vi "Dashboard Main_1366_768.vi"() -> ()   [LabVIEW 2020]
uses:
  ArmGamePiecePreset.ctl
  ArmPositionPreset.ctl
  <vilib>/Rock Robotics/WPI/ThirdParty/JAS_Junk/TrajLib/TypeDef/FieldDisp_ElementPicture.ctl
  <vilib>/Rock Robotics/WPI/Solenoid/WPI_SolenoidValue.ctl
  <vilib>/event_ctls.llb/eventvkey.ctl
  <vilib>/Rock Robotics/WPI/ThirdParty/JAS_Junk/TrajLib/Rotation2d_CreateAngle.vi
  <vilib>/Rock Robotics/WPI/ThirdParty/JAS_Junk/TrajLib/Translation2d_Create.vi
  <vilib>/Rock Robotics/WPI/ThirdParty/JAS_Junk/TrajLib/VI/FieldDisp_Element_Rotate.vi
  <vilib>/Rock Robotics/WPI/ThirdParty/JAS_Junk/TrajLib/Conv_Meters_Inches.vi
  <vilib>/Rock Robotics/WPI/ThirdParty/JAS_Junk/TrajLib/Conv_Radians_Deg.vi
  <vilib>/Rock Robotics/WPI/Dashboard/WPI_DashboardLogging Global.vi
  <vilib>/Rock Robotics/Network Tables/NT Read Boolean.vi
  <vilib>/Rock Robotics/Network Tables/NT Read Integer.vi
  <vilib>/picture/pixmap.llb/Flatten Pixmap.vi
  <vilib>/picture/pictutil.llb/Create Mask.vi
  <vilib>/picture/picture.llb/Draw Flattened Pixmap.vi
  <vilib>/Rock Robotics/WPI/ThirdParty/JAS_Junk/TrajLib/Trajectory_Library.lvlib
panel:
  out "ROBOT":T1
  out "Camera Perf":string
  in  "Camera Settings":T2={"Frame Rate"=30, "Compression"=30, "Size"=1, "DB Camera Config"=FALSE} {"Frame Rate" scale=1.0..30.0; "Compression" scale=100.0..-1.0; "Size" items=["640x480", "320x240", "160x120"]}
  in  "TCP":refnum<k5>
  in  "Rec Mode":enum32{"Stop", "Record", "Playback"}(radio)
  out "Robot IP":string
  out "Image Message":string="Timeout in Camera Communications"
  in  "Dashboard Tab":T3(tab)
  out "Double Cmd1":T4
  out "Double Cmd2":T4
  out "Single Cmd1":T4
  out "Single Cmd2":T4
  out "Request":bool
  out "On Command":bool
  out "On Command":bool
  out "Request":bool
  out "Current":dbl format="%12.2f"
  out "Running":bool
  out "Enabled":bool
  out "NT Connection":bool
  out "Mode":T5(ring)=enum."Auto Disabled"
  out "Right Camera Perf":cluster{"Bandwidth (Mbps)":dbl, "FPS":dbl}
  out "Shelf":bool
  out "Floor":bool
  out "Right April Tag Updated":bool
  out "Left April Tag Updated":bool
  out "Right Cam Connected":bool
  out "Left Cam Connected":bool
  out "Field Picture":picture
  out "Odom X Pos Ft":dbl format="%14.2f"
  out "Odom Y Pos Ft":dbl format="%14.2f"
  out "Odom Heading Deg":dbl format="%14.2f"
  in  "Distance":dbl
  in  "Position":T6=enum."Middle"
  in  "Game Piece":T7
  in  "Update":bool
  in  "Starting Heading Deg":dbl
  in  "Starting Y Ft":dbl
  in  "Starting X Ft":dbl
  in  "DB/String 9":string
  in  "DB/String 8":string
  in  "DB/String 7":string
  in  "DB/String 6":string
  in  "DB/String 5":string
  in  "DB/String 4":string
  in  "DB/String 3":string
  in  "DB/String 2":string
  in  "DB/String 1":string
  in  "DB/String 0":string
  in  "DB/Slider 0":dbl(slide) scale=0.0..5.0
  in  "DB/Slider 1":dbl(slide) scale=0.0..5.0
  in  "DB/Slider 2":dbl(slide) scale=0.0..5.0
  in  "DB/Slider 3":dbl(slide) scale=0.0..5.0
  out "DB/LED 3":bool
  out "DB/LED 2":bool
  out "DB/LED 1":bool
  out "DB/LED 0":bool
  in  "DB/Button 3":bool
  in  "DB/Button 2":bool
  in  "DB/Button 1":bool
  in  "DB/Button 0":bool caption="New Name"
  out "Compressor Chart":cluster{"value":dbl, "value":dbl, "value":dbl}(graph)
  out "Single Solenoid Chart":cluster{"value":dbl, "value":dbl, "value":dbl}(graph)
  out "Double Solenoid Chart":cluster{"value":dbl, "value":dbl, "value":dbl}(graph)
  in  "Test Slider":dbl(slide) scale=0.0..100.0 scale format="%#_3g"
  in  "On/Off":bool caption="Solenoid"
  in  "Test Name":u16(ring) items=["Select the test to run..."]
  in  "Test Tree":string(tree)
  in  "Motor":cluster{"Value":dbl, "Enable":bool} {"Value" scale=-1.0..1.0 scale format="%#_3g"}
  out "Progress":T8 {"Test Progress" scale=0.0..100.0}
  in  "Rev/Fwd":cluster{"Forward":bool, "Reverse":bool}
  in  "Test Ring":u16(ring) items=["Monochrome", "Color"]
  in  "CheckList":i32(listbox)
  out "Tree":string(tree)
  out "Camera Image":T9(plugin-control)
  out "Background":bool
  in  "Camera Name":string(combo)="No Camera Selection"
  # "HW"
  # "Double Solenoid"
  # "Single Solenoid"
  # "Compressor"
  # "Quick Auto Settings"
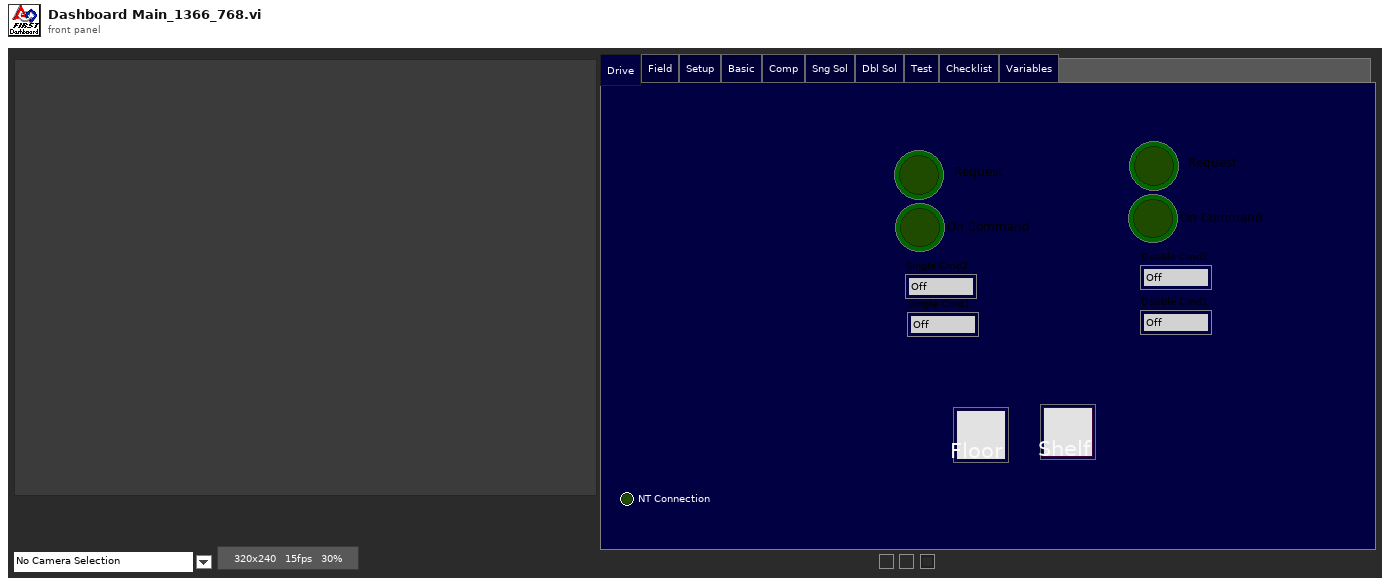
[diagram p1: front panel]
types:
  T1 = typedef "Trajectory_Library.lvlib/FieldDisp_ElementPicture.ctl" = picture
  T2 = cluster{"Frame Rate":i32, "Compression":i32, "Size":u16, "DB Camera Config":bool}
  T3 = enum32{"Drive", "Field", "Setup", "Basic", "Comp", "Sng Sol", "Dbl Sol", "Test", "Checklist", "Variables"}
  T4 = typedef "WPI_SolenoidValue.ctl" = enum16{"Off", "On", "Forward", "Reverse"}
  T5 = enum8{"Tele-Op Disabled", "Tele-Op Enabled", "Auto Disabled", "Auto Enabled", "Test Disabled", "Test Enabled", "Disconnected", "No Code", "E-Stop"}
  T6 = typedef "ArmPositionPreset.ctl" = enum16{"Upper", "Lower", "Middle", "Home", "Shelf", "Floor"}
  T7 = typedef "ArmGamePiecePreset.ctl" = enum16{"Cube", "Cone"}
  T8 = cluster{"Test Progress":u8, "Test Progress Text":string}
  T9 = typedef "IMAQ Image.ctl" = refnum<image>
  T10 = enum32{"Drive", "Field", "Setup", "Basic", "DrvLeft", "DrvRight", "ArmExtend", "ArmLift", "Bal", "Test", "Checklist", "Variables"}
  T11 = cluster{"Save Path":path, "Interval (s)":dbl, "Keep":i32}
  T12 = typedef "Image Type" = u32
  T13 = cluster{"Camera Image":refnum<vi>, "Dashboard Tab":refnum<vi>, "Background":refnum<vi>, "Rec Mode":refnum<vi>, "Test Slider":refnum<vi>, "On/Off ":refnum<vi>, "Test Ring":refnum<vi>, "Rev/Fwd":refnum<vi>, "Test Name":refnum<vi>, "Motor":refnum<vi>, "Progress":refnum<vi>, "CheckList":refnum<vi>, "Tree":refnum<vi>, "Test Tree":refnum<vi>, "Camera Settings":refnum<vi>, "Camera Name":refnum<vi>, "Camera Perf":refnum<vi>}
  T14 = cluster{"Global Rectangle":i32[], "Contours":cluster{"Contour Type":u32, "ROI Type":u32, "Points":i32[]}[]}
  T15 = cluster{"Camera Name":string, string, "Saved DB Images Info":cluster{"Save Path":path, "Interval (s)":dbl, "Keep":i32}}
  T16 = cluster{"Operation":enum16{"Update", "Clear"}, "Color Box":u32}[]
  T17 = typedef "eventvkey.ctl" = enum16{"ASCII", "Enter", "Return", "Shift", "Ctrl", "Alt", "Cmd", "Opt", "Caps", "NumLock", "Clear", "Break", "Up", "Down", "Left", "Right", "Insert", "Delete", "Home", "End", "PageUp", "PageDown", "Escape", "Help", "Pause", "ScrollLock", "F1", "F2", "F3", "F4", "F5", "F6", "F7", "F8", "F9", "F10", "F11", "F12", "F13", "F14", "F15", "F16", "F17", "F18", "F19", "F20", "F21", "F22", "F23", "F24", "Play", "VolumeUp", "VolumeDown", "Mute", "Two Byte Char"}
  T18 = cluster{"Image Size":bool, "Image Type":bool, "Pixel Value":bool, "ROI Information":bool, "Zoom Factor":bool}
  T19 = cluster{"Operation":enum16{"Update", "Clear"}, "Color Box":u32}
  T20 = cluster{"Shift":bool, "Ctrl":bool, "Alt":bool, "Cmd":bool, "Opt":bool}
  T21 = typedef "Trajectory_Library.lvlib/FieldDisp_FieldElement.ctl" = cluster{"ONE-8-bit pixmap":u8[][], "Two-Array":cdb[][], "Three-Numeric":i32, "Four-Numeric":i32, "Five-Numeric":cdb, "Six-colors":u32[], "Seven-new element/subarray":u32, "Left Poxel":dbl, "Top Pixel":dbl, "Width Pix/Ft":dbl, "Height Pix/Ft":dbl, "Element Picture Ref":refnum<vi>}
  T22 = cluster{"Error Strings":string, "Disable Counts":cluster{u16, u16}, "Rail Faults":cluster{u16, u16, u16}, "Robot IP":string, "DB Mode":u8, "Event Info":cluster{"Name":string, "Type":u8, "Number":u16, "Replay":u8}}
  T23 = cluster{"Storage":cluster{"Disk Free":u64, "RAM Block":u32, "RAM free":u32}, "CPU Utilization":cluster{"CPU % ISR":sgl, "CPU % Time Crit":sgl, "CPU % Timed Str":sgl, "CPU % High":sgl, "CPU % Above":sgl, "CPU % Normal":sgl, "CPU % Low":sgl}, "CAN":cluster{"% Bus Utilization":sgl, "Bus Off Cnt":u32, "TX_FIFO Full Cnt":u32, "Receive Error Cnt":u8, "Transmit Error Cnt":u8}, "HID":cluster{"HID Outputs":u32, "Rumble Low":u16, "Rumble High":u16}[]}
  T24 = cluster{"Status bits":cluster{"Test Mode":bool, "Autonomous":bool, "Enabled":bool, "Code Start":bool, "Brownout":bool, "Reserved 2":bool, "Reserved 3":bool, "E-Stop":bool}, "Code Trace":cluster{"Disabled":bool, "TeleOp":bool, "Auto":bool, "Test":bool}, "Controller Type":enum16{"unknown", "cRIO", "roboRio"}, "Code?":enum16{"unknown", "noCode", "code"}, "Battery V":dbl}
  T25 = cluster{"Control Bits":cluster{"TestMode":bool, "Autonomous":bool, "Enabled":bool, "FMS Present":bool, bool, bool, bool, "E-Stop":bool}, "Team Station ":u8, "Countdown":sgl, "Joystick Values":cluster{"Axes":dbl[], "Buttons":bool[], "POVs":i16[]}[]}
  T26 = typedef "Trajectory_Library.lvlib/POSE2D.ctl" = cluster{"TRANSLATION":T27, "ROTATION":T28}
  T27 = typedef "Trajectory_Library.lvlib/TRANSLATION2D.ctl" = cluster{"X":dbl, "Y":dbl}
  T28 = typedef "Trajectory_Library.lvlib/ROTATION2D.ctl" = cluster{"VALUE":dbl, "COS":dbl, "SIN":dbl}
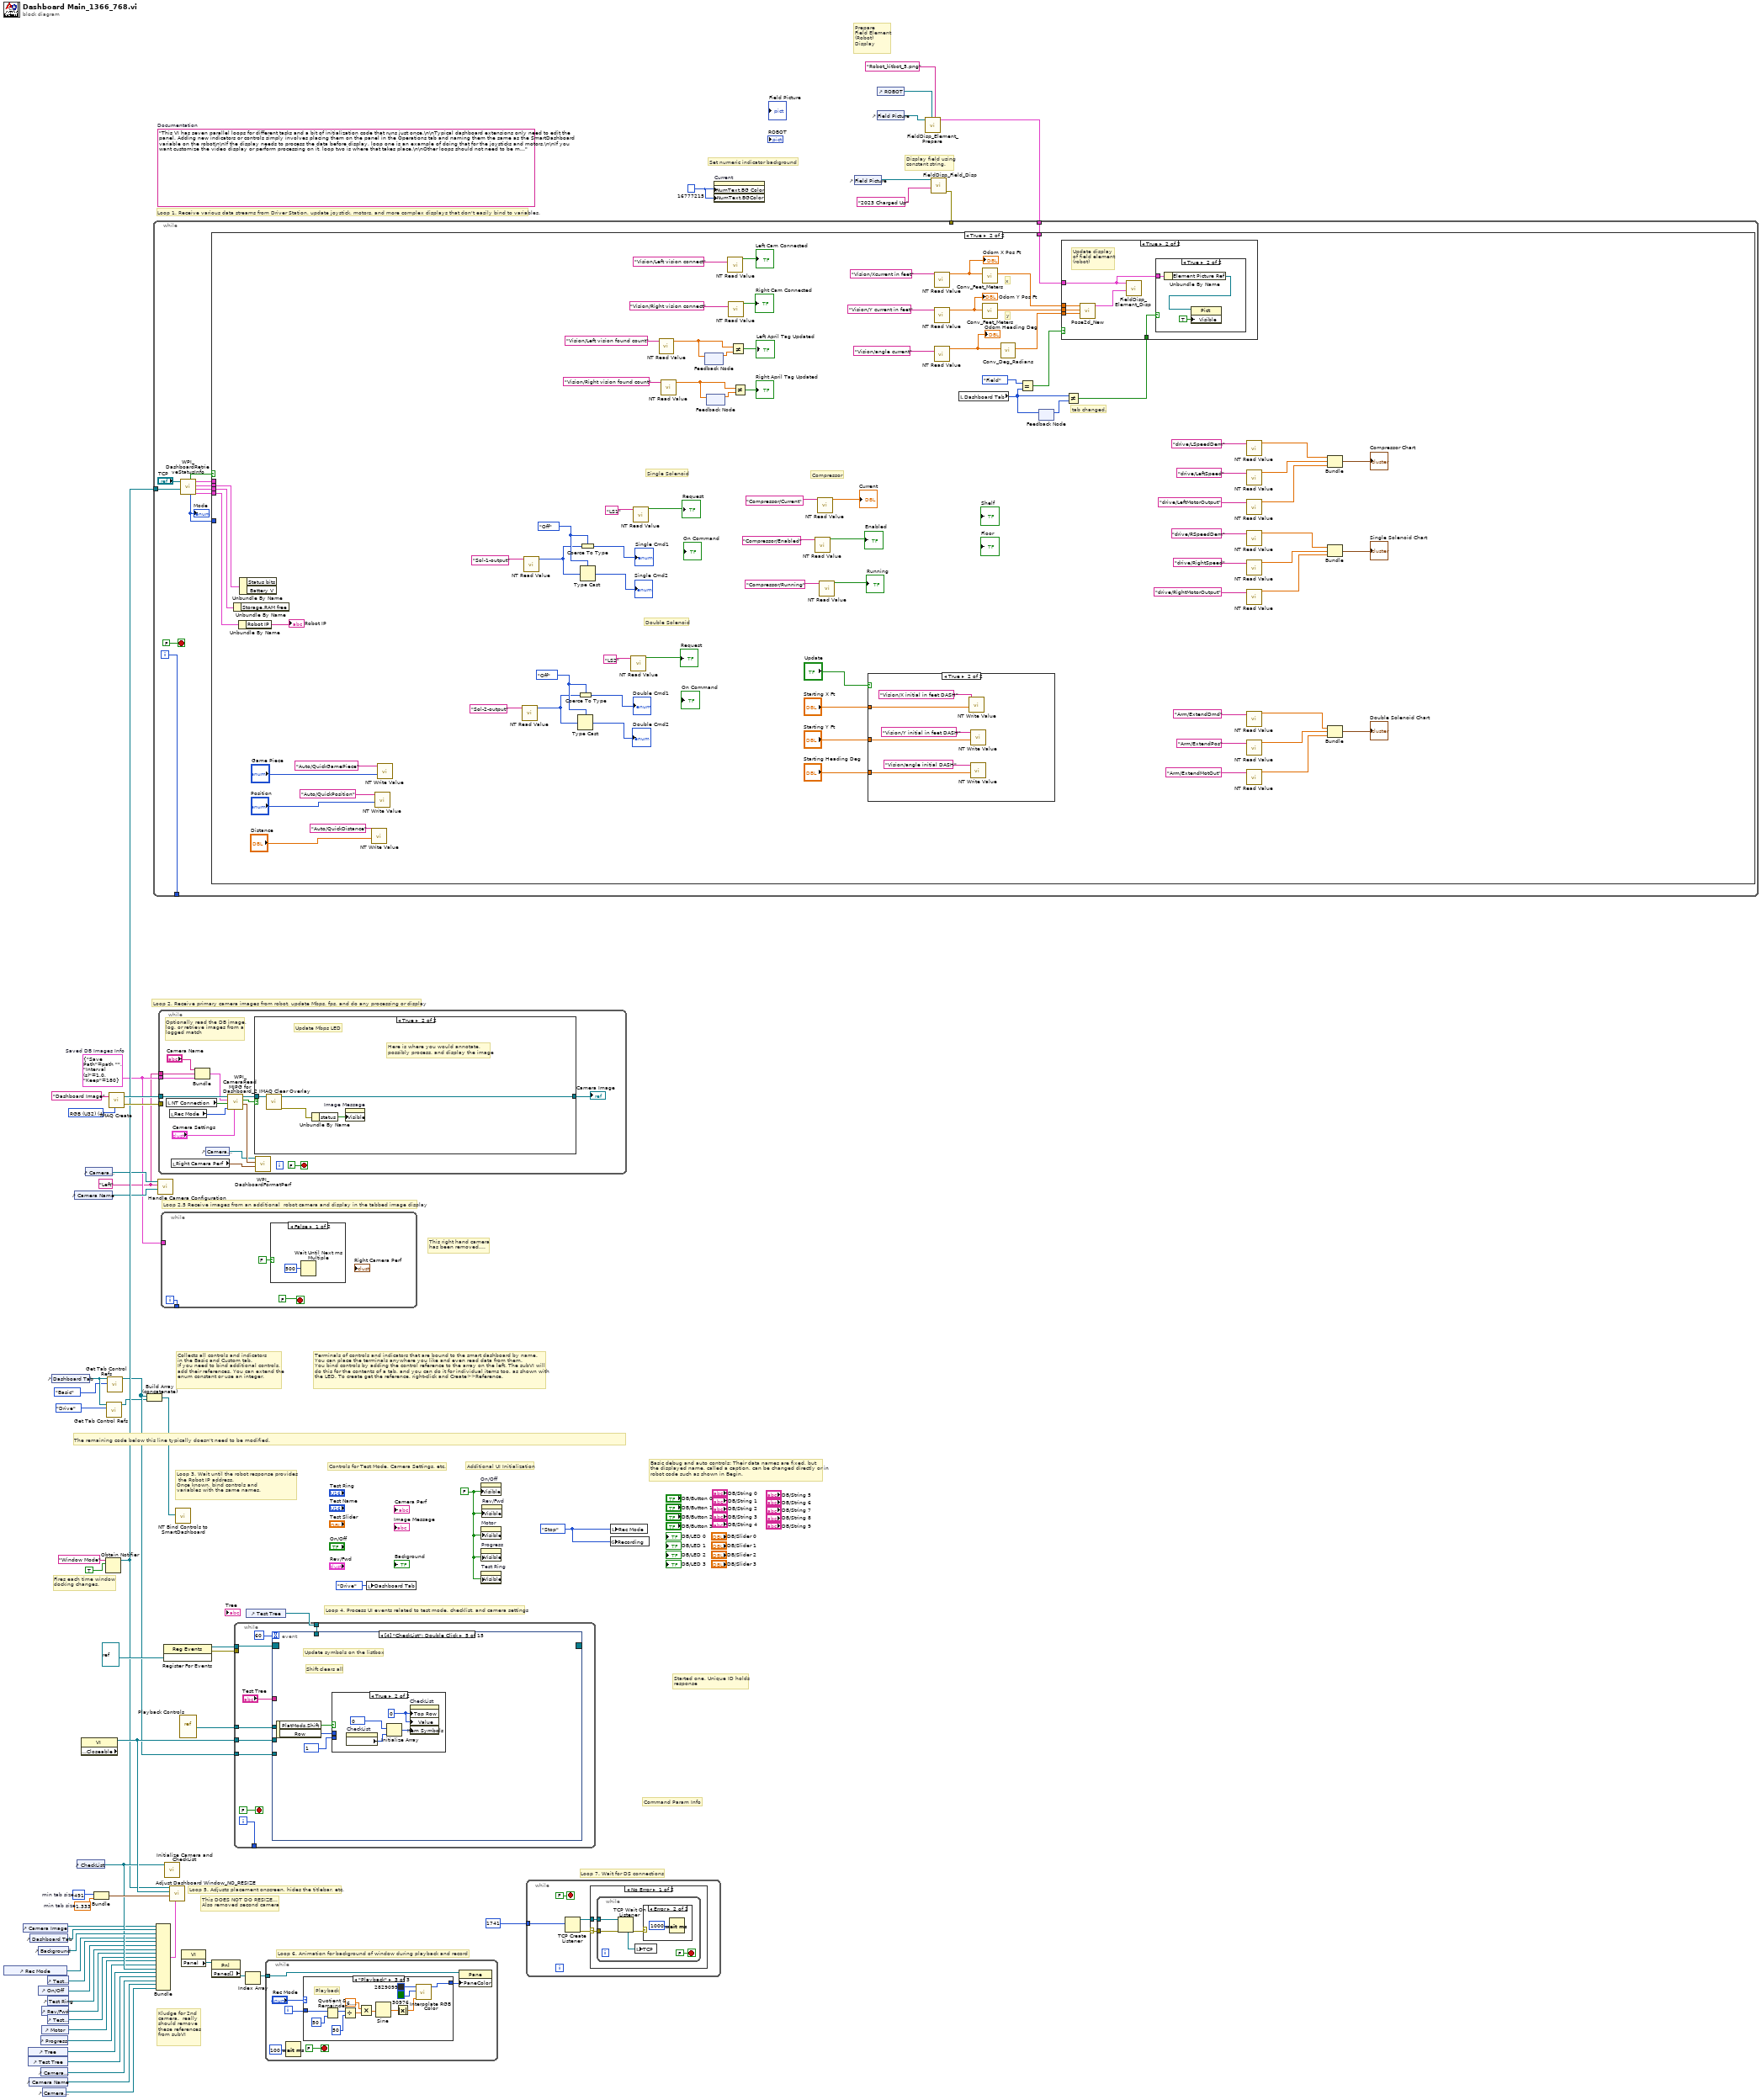
[diagram p0: block diagram]
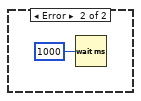
[diagram p4: hidden frame]
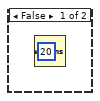
[diagram p5: hidden frame]
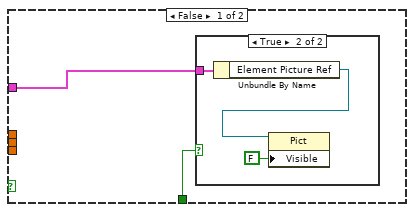
[diagram p6: hidden frame]
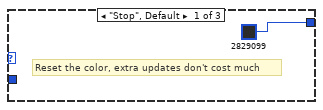
[diagram p10: hidden frame]
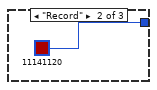
[diagram p11: hidden frame]
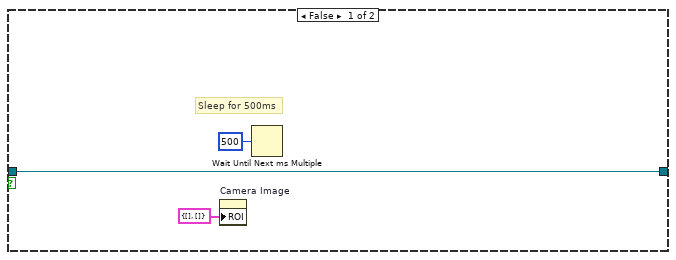
[diagram p12: hidden frame]
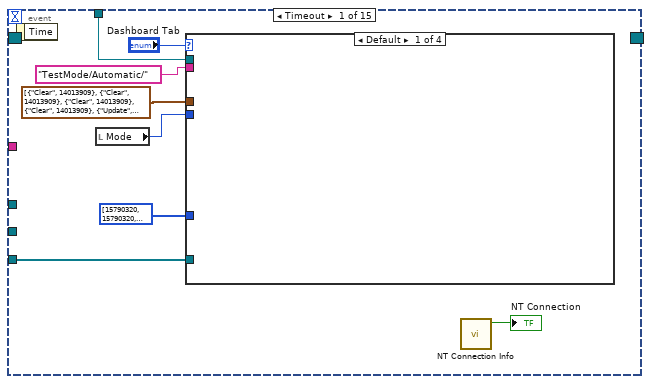
[diagram p13: hidden frame]
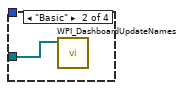
[diagram p14: hidden frame]
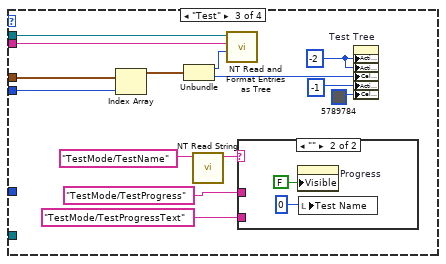
[diagram p15: hidden frame]
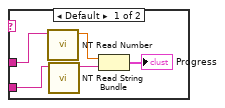
[diagram p16: hidden frame]
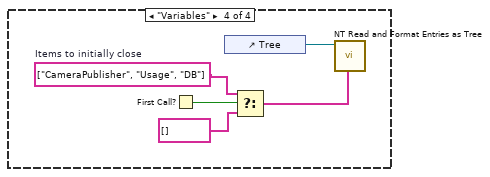
[diagram p17: hidden frame]
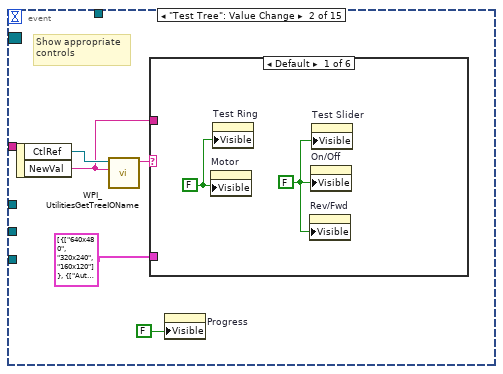
[diagram p18: hidden frame]
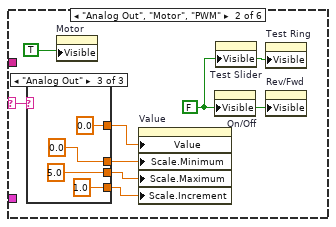
[diagram p19: hidden frame]
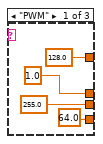
[diagram p20: hidden frame]
diagram:
  w2 = u32 16777215 ("Caption.Colors:BG Color")
  w18 = T11 {"Save Path"=path "", "Interval (s)"=1.0, "Keep"=180}  # Saved DB Images Info
  w17 = "Left"
  w41 = 491  # min tab size
  w40 = 1.333  # min tab size
  w45 = enum32{"Stop", "Record", "Playback"}."Stop" ("Rec Mode")
  w25 = FALSE ("Visible")
  (unwired) "This VI has seven parallel loops for different tasks and a bit of initialization code that runs just once.\n\nTypical dashboard extensions only need to edit the panel. Adding new indicators or controls simply involves placing them on the panel in the Operations tab and naming them the same as the SmartDashboard variable on the robot\n\nIf the display needs to process the data before display, loop one is an example of doing that for the joysticks and motors.\n\nIf you want customize the video display or perform processing on it, loop two is where that takes place.\n\nOther loops should not need to be modified. They are pretty standard, and document the task they perform."  # Documentation
  w59 = T12 4 items=["Grayscale (U8)", "Grayscale (I16)", "Grayscale (SGL)", "Complex (CSG)", "RGB (U32)", "HSL (U32)", "RGB (U64)"] ("Image Type")
  # "Set numeric indicator background"
  # "Display field using\nconstant string."
  # "Prepare\nField Element\n(Robot)\nDisplay"
  # "Kludge for 2nd\ncamera.  really\nshould remove\nthese references\nfrom subVI"
  # "This right hand camera\nhas been removed...."
  # "This DOES NOT DO RESIZE...\nAlso removed second camera"
  # "Loop 2.5 Receive images from an additional  robot camera and display in the tabbed image display"
  # "Command Param Info"
  # "Started one, Unique ID holds\nresponse"
  # "Loop 7. Wait for DS connections"
  # "Basic debug and auto controls: Their data names are fixed, but\nthe displayed name, called a caption, can be changed directly or in\nrobot code such as shown in Begin."
  # "Controls for Test Mode, Camera Settings, etc."
  # "Additional UI Initialization"
  # "Loop 6. Animation for background of window during playback and record"
  # "Fires each time window\ndocking changes."
  # "Collects all controls and indicators\nin the Basic and Custom tab.\nIf you need to bind additional controls,\nadd their references. You can extend the\nenum constant or use an integer."
  # "The remaining code below this line typically doesn't need to be modified."
  # "Loop 4. Process UI events related to test mode, checklist, and camera settings"
  # "Terminals of controls and indicators that are bound to the smart dashboard by name.\nYou can place the terminals anywhere you like and even read data from them.\nYou bind controls by adding the control reference to the array on the left. The subVI will\ndo this for the contents of a tab, and you can do it for individual items too, as shown with\nthe LED. To create get the reference, right-click and Create>>Reference."
  # "Loop 3. Wait until the robot response provides\n the Robot IP address.\nOnce known, bind controls and\nvariables with the same names."
  # "Loop 5. Adjusts placement onscreen, hides the titlebar, etc."
  # "Loop 1. Receive various data streams from Driver Station, update joystick, motors, and more complex displays that don't easily bind to variables."
  # "Loop 2. Receive primary camera images from robot, update Mbps, fps, and do any processing or display"
  n1 = control-ref of="Rec Mode"() -> (w31:refnum<vi>)
  n2 = control-ref of="Camera Image"() -> (w14:refnum<vi>)
  n3 = control-ref of="Tree"() -> (w35:refnum<vi>)
  n4 = control-ref of="Test Tree"() -> (w34:refnum<vi>)
  n5 = control-ref of="Camera Name"() -> (w15:refnum<vi>)
  n6 = control-ref of="Dashboard Tab"() -> (w42:refnum<vi>)
  n7 = control-ref of="Background"() -> (w38:refnum<vi>)
  n8 = control-ref of="On/Off"() -> (w29:refnum<vi>)
  n9 = control-ref of="Progress"() -> (w26:refnum<vi>)
  n10 = control-ref of="Camera Settings"() -> (w16:refnum<vi>)
  n11 = control-ref of="Rev/Fwd"() -> (w27:refnum<vi>)
  n12 = control-ref of="Motor"() -> (w32:refnum<vi>)
  n13 = control-ref of="Camera Perf"() -> (w20:refnum<vi>)
  n14 = control-ref of="Test Slider"() -> (w30:refnum<vi>)
  n15 = control-ref of="Test Ring"() -> (w28:refnum<vi>)
  n16 = control-ref of="Test Name"() -> (w33:refnum<vi>)
  n17 = control-ref of="Dashboard Tab"() -> (w6:refnum<vi>)
  n18 = control-ref of="Camera Name"() -> (w21:refnum<vi>)
  n19 = control-ref of="CheckList"() -> (w36:refnum<vi>)
  n20 = property class="VI" props=["Front Panel.Closeable"]() -> (reference out=w44:refnum<vi>)  [unwired: 2 in, 2 out]
  n21 = control-ref of="Camera Settings"() -> (w22:refnum<vi>)
  n22 = Bundle("min tab size"=w41, "min tab size"=w40) -> (w39:cluster{"min tab size":i32, "min tab size":dbl})  [unwired: 1 in]
  n23 = Obtain Notifier(name (unnamed)="Window Mode", notification data type=TRUE) -> (notifier out=w24:refnum<notifier>)  [unwired: 2 in, 2 out]
  n24 = call <vilib>:"Get Tab Control Refs.vi"("Page Index"=T10."Drive" ("Dashboard Tab"), "TabControl in"=w6) -> ("ControlsOnPage"=w7:refnum<vi>[])  [unwired: 9 in]
  n25 = call <vilib>:"Get Tab Control Refs.vi"("Page Index"=T10."Basic" ("Dashboard Tab"), "TabControl in"=w6) -> ("ControlsOnPage"=w19:refnum<vi>[])  [unwired: 9 in]
  n26 = call "IMAQ Create"("Image Name"="Dashboard Image", "Image Type"=w59) -> ("New Image"=w57:T9, "error out"=w56:errorcluster)  [unwired: 2 in, 1 out]
  n27 = Build Array (concatenate)(w19, w7) -> (w43:refnum<vi>[])
  n28 = Bundle("Camera Image"=w14, "Dashboard Tab"=w42, "Background"=w38, "Rec Mode"=w31, "Test Slider"=w30, "On/Off"=w29, "Test Ring"=w28, "Rev/Fwd"=w27, "Test Name"=w33, "Motor"=w32, "Progress"=w26, "CheckList"=w36, "Tree"=w35, "Test Tree"=w34, "Camera Settings"=w16, "Camera Name"=w15, "Camera Perf"=w20) -> (w37:T13)  [unwired: 1 in]
  n29 = call "Handle Camera Configuration.vi"("CameraNameRef"=w21, "Display Name"=w17, "ClusterRef"=w22) -> ()  [unwired: 9 in]
  n30 = while {
    tunnel: w57 -> [w73]
    tunnel: w56 -> [_]
    tunnel: w18 -> [w66]
    tunnel: w17 -> [w63]
    stop <- FALSE stop-if-true
    # "Optionally read the DB image,\nlog, or retrieve images from a\nlogged match"
    n31 = local read "NT Connection"() -> (w67:bool)
    n32 = local read "Rec Mode"() -> (w70:enum32{"Stop", "Record", "Playback"})
    n33 = local read "Right Camera Perf"() -> (w61:cluster{"Bandwidth (Mbps)":dbl, "FPS":dbl})
    n34 = Bundle("Camera Name"="Camera Name", w63, "Saved DB Images Info"=w66) -> (w65:T15)  [unwired: 1 in]
    n35 = control-ref of="Camera Perf"() -> (w60:refnum<vi>)
    n36 = call <vilib>:"WPI_CameraRead MJPG for Dashboard_2.vi"("Camera Settings"="Camera Settings", "Rec Mode"=w70, "NT Connection"=w67, "Capture Info"=w65, "Image in"=w73) -> ("perf info"=w62:cluster{"Bandwidth (Mbps)":dbl, "fps":dbl}, "Active"=w71:bool, "Image\\ out"=w72:T9)  [unwired: 4 in]
    n37 = case shown="True" w71 {
      tunnel: w72 -> [w76 w79]
      tunnel: [w76 w78] -> w68
      frame False {
        # "Sleep for 500ms"
        n38 = property on="Camera Image" class="ImageControl"("ROI"=T14 {"Global Rectangle"=[], "Contours"=[]}) -> ()  [unwired: 2 in, 2 out]
        n39 = Wait Until Next ms Multiple(millisecond multiple=u32 500) -> ()  [unwired: 1 out]
      }
      frame True {
        # "Here is where you would annotate,\npossibly process, and display the image"
        # "Update Mbps LED"
        n40 = call "IMAQ Clear Overlay"("Image"=w79) -> ("error out"=w80:errorcluster, "Image Out"=w78:T9)  [unwired: 2 in, 7 out]
        n41 = Unbundle By Name(w80) -> ("status"=w81:bool)
        n42 = property on="Image Message" class="Str"("Visible"=w81) -> ()  [unwired: 2 in, 2 out]
      }
    }
    "Camera Image" <- w68
    n43 = call <vilib>:"WPI_DashboardFormatPerf.vi"("Right Camera Perf"=w61, "Performance"=w62, "String in"=w60) -> ()  [unwired: 9 in]
  }
  n44 = while {
    tunnel: [w83] -> _
    tunnel: w18 -> [_]
    i -> [w83]
    stop <- FALSE stop-if-true
    n45 = case shown="False" FALSE {
      frame False {
        n46 = Wait Until Next ms Multiple(millisecond multiple=u32 500) -> ()  [unwired: 1 out]
      }
      frame True {
      }
    }
  }
  n47 = register-events(refnum<vi> refnum) -> (reference out=w48:refnum<event-registration>, error out=w47:errorcluster)  [unwired: 2 in]
  n48 = call "Initialize Camera and CheckList.vi"("ListBox in"=w36) -> ()  [unwired: 11 in]
  n49 = call "Adjust Dashboard Window_NO_RESIZE.vi"("Sizing Refnums"=w37, "Size Constraints"=w39, "VI"=w44, "WIn Mode"=w24) -> ()  [unwired: 8 in]
  n50 = call <vilib>:"NT Bind Controls to SmartDashboard.vi"("Bound Control Refs"=w43) -> ()  [unwired: 11 in]
  n51 = vi-ref "Playback Controls.vi"() -> (w49:refnum<vi>)
  n52 = property class="VI"() -> ("Panel"=w51:refnum<vi>)  [unwired: 2 in, 2 out]
  n53 = property class="Pnl"(reference=w51) -> ("Panes[]"=w52:refnum<vi>[])  [unwired: 1 in, 2 out]
  n54 = Index Array(array=w52) -> (element=w50:refnum<vi>)  [unwired: 1 in]
  n55 = control-ref of="Test Tree"() -> (w53:refnum<vi>)
  n56 = while {
    tunnel: [w91] -> _
    tunnel: w53 -> [w90]
    tunnel: w49 -> [w89]
    tunnel: w48 -> [w88]
    tunnel: w47 -> [_]
    tunnel: w44 -> [w87]
    tunnel: w19 -> [w86]
    i -> [w91]
    stop <- FALSE stop-if-true
    n57 = event shown="[4] \"CheckList\": Double Click" {
      selector: w88 -> [_ _ _ _ _ _ _ _ _ _ _ _ _ _ _]
      dyn-events: [_ _ _ _ _ _ _ _ _ _ _ w292 _ _ _] -> _
      timeout: u32 60 ("milliseconds to wait") -> [_ _ _ _ _ _ _ _ _ _ _ _ _ _ _]
      tunnel: w90 -> [w101 _ _ _ _ _ _ _ _ _ _ _ _ _ _]
      tunnel: "Test Tree" -> [_ _ _ _ _ _ w265 w272 w273 w276 w283 _ _ _ _]
      tunnel: w89 -> [_ _ _ _ _ _ _ _ _ _ _ w294 _ w309 _]
      tunnel: w87 -> [_ _ _ _ _ _ _ _ _ _ _ w290 _ _ _]
      tunnel: w86 -> [w96 _ _ _ _ _ _ _ _ _ _ _ _ _ _]
      event Timeout {
        n58 = event-data() -> ()  [unwired: 1 in, 1 out]
        n59 = local read "Mode"() -> (w99:T5)
        n60 = case shown="Default" "Dashboard Tab" {
          tunnel: w101 -> [_ _ w117 _]
          tunnel: "TestMode/Automatic/" ("Name Pattern") -> [_ _ w116 _]
          tunnel: T16 [{"Operation"=enum."Clear", "Color Box"=14013909}, {"Operation"=enum."Clear", "Color Box"=14013909}, {"Operation"=enum."Clear", "Color Box"=14013909}, {"Operation"=enum."Clear", "Color Box"=14013909}, {"Operation"=enum."Update", "Color Box"=14013909}, {"Operation"=enum."Update", "Color Box"=16777215}, {"Operation"=enum."Clear", "Color Box"=14013909}, {"Operation"=enum."Clear", "Color Box"=14013909}, {"Operation"=enum."Clear", "Color Box"=14013909}] -> [_ _ w109 _]
          tunnel: w99 -> [_ _ w108 _]
          tunnel: u32[] [15790320, 15790320, 15790320, 15790320, 16777215, 16777215, 15790320, 15790320, 15790320] -> [_ _ _ _]
          tunnel: w96 -> [_ w103 _ _]
          frame Default {
          }
          frame "Basic" {
            n61 = call <vilib>:"WPI_DashboardUpdateNames.vi"("Controls on Tab"=w103) -> ()  [unwired: 11 in]
          }
          frame "Test" {
            w115 = -2 ("Active Item:Row Number")
            n62 = Index Array(array=w109, index=w108) -> (element=w110:T19)
            n63 = Unbundle(w110) -> ("Operation"=w111:enum16{"Update", "Clear"}, "Color Box"=w112:u32)
            n64 = call <vilib>:"NT Read String.vi"("name"="TestMode/TestName" ("Name")) -> ("value"=w106:string)  [unwired: 8 in, 2 out]
            n65 = call <vilib>:"NT Read and Format Entries as Tree.vi"("Operation"=w111, "Name Pattern"=w116, "Tree Refnum"=w117) -> ()  [unwired: 7 in, 2 out]
            n66 = case shown="\"\"" w106 {
              tunnel: "TestMode/TestProgress" ("Name") -> [w119 _]
              tunnel: "TestMode/TestProgressText" ("Name") -> [w118 _]
              frame Default {
                n67 = call <vilib>:"NT Read Number.vi"("name"=w119) -> ("value"=w120:dbl)  [unwired: 8 in, 2 out]
                n68 = call <vilib>:"NT Read String.vi"("name"=w118) -> ("value"=w121:string)  [unwired: 8 in, 2 out]
                n69 = Bundle("value"=w120, "value"=w121) -> (→"Progress":cluster{"value":dbl, "value":string})  [unwired: 1 in]
              }
              frame "" {
                n70 = property on="Progress" class="Clust (strict)"("Visible"=FALSE) -> ()  [unwired: 2 in, 2 out]
                n71 = local write "Test Name"(u16 0) -> ()
              }
            }
            n72 = property on="Test Tree" class="Tree (strict)"("Active Item Row Number"=w115, "ActiveColNum"=w115, "CellBG"=w112, "Active Item Row Number"=-1 ("Active Item:Row Number"), "CellBG"=u32 5789784 ("Color Box")) -> ()  [unwired: 2 in, 2 out]
          }
          frame "Variables" {
            w127 = string[] ["CameraPublisher", "Usage", "DB"]  # Items to initially close
            n73 = First Call?() -> (First Call?: T/F=w128:bool)
            n74 = control-ref of="Tree"() -> (w129:refnum<vi>)
            n75 = Select(t=w127, s=w128, f=string[] []) -> (s? t:f=w125:string[])
            n76 = call <vilib>:"NT Read and Format Entries as Tree.vi"("Tags to  Close"=w125, "Tree Refnum"=w129) -> ()  [unwired: 8 in, 2 out]
          }
        }
        n77 = call <vilib>:"NT Connection Info.vi"() -> ("Connected"=→"NT Connection":bool)  [unwired: 11 in]
      }
      event "Test Tree": Value Change {
        # "Show appropriate\ncontrols"
        n78 = event-data() -> ("CtlRef"=w133:refnum<vi>, "NewVal"=w131:string)  [unwired: 1 in]
        n79 = call <vilib>:"WPI_UtilitiesGetTreeIOName.vi"("NewVal"=w131, "TreeControl in"=w133) -> ("I/O Name"=w134:string)  [unwired: 9 in]
        n80 = case shown="Default" w134 {
          selector: w134 -> [_ w141 _ w163 w172 _]
          tunnel: w131 -> [_ _ w160 w162 _ w179]
          tunnel: cluster{string[]}[] [{["640x480", "320x240", "160x120"]}, {["Auto", "Fixed indoor", "Fixed outdoor 1", "Fixed outdoor 2", "Fixed fluorescent 1", "Fixed fluorescent 2", "Hold current"]}, {["Auto", "Flicker-free 50 Hz", "Flicker-free 60 Hz", "Hold current"]}, {["None", "Prioritize frame rate", "Prioritize image quality"]}, {["Monochrome", "Color"]}] -> [_ _ _ _ _ w178]
          frame Default {
            w136 = FALSE ("Visible")
            w135 = FALSE ("Visible")
            n81 = property on="Motor" class="Clust (strict)"("Visible"=w135) -> ()  [unwired: 2 in, 2 out]
            n82 = property on="Test Ring" class="Ring (strict)"("Visible"=w135) -> ()  [unwired: 2 in, 2 out]
            n83 = property on="Rev/Fwd" class="Clust (strict)"("Visible"=w136) -> ()  [unwired: 2 in, 2 out]
            n84 = property on="On/Off" class="Bool (strict)"("Visible"=w136) -> ()  [unwired: 2 in, 2 out]
            n85 = property on="Test Slider" class="Slide (strict)"("Visible"=w136) -> ()  [unwired: 2 in, 2 out]
          }
          frame "Analog Out", "Motor", "PWM" {
            w142 = FALSE ("Visible")
            n86 = case shown="\"Analog Out\"" w141 {
              tunnel: [1.0 ("Value") -1.0 ("Value") 0.0 ("Value")] -> w140
              tunnel: [255.0 ("Value") 1.0 ("Value") 5.0 ("Value")] -> w139
              tunnel: [128.0 ("Value") 0.0 ("Value") 0.0 ("Value")] -> w138
              tunnel: [64.0 ("Value") 0.5 ("Value") 1.0 ("Value")] -> w137
              frame "PWM" {
              }
              frame "Motor", Default {
              }
              frame "Analog Out" {
              }
            }
            n87 = property on="Motor" class="Clust (strict)"("Visible"=TRUE) -> ()  [unwired: 2 in, 2 out]
            n88 = property on="Value" class="Slide (strict)"("Value"=w138, "Scale.Minimum"=w140, "Scale.Maximum"=w139, "Scale.Increment"=w137) -> ()  [unwired: 2 in, 2 out]
            n89 = property on="On/Off" class="Bool (strict)"("Visible"=w142) -> ()  [unwired: 2 in, 2 out]
            n90 = property on="Test Slider" class="Slide (strict)"("Visible"=w142) -> ()  [unwired: 2 in, 2 out]
            n91 = property on="Test Ring" class="Ring (strict)"("Visible"=w142) -> ()  [unwired: 2 in, 2 out]
            n92 = property on="Rev/Fwd" class="Clust (strict)"("Visible"=w142) -> ()  [unwired: 2 in, 2 out]
          }
          frame "Servo" {
            w158 = FALSE ("Visible")
            n93 = call <vilib>:"NT Read Number.vi"("name"=w160) -> ("value"=w159:dbl)  [unwired: 8 in, 2 out]
            n94 = property on="Test Slider" class="Slide (strict)"("Visible"=TRUE, "Scale.Maximum"=170.0 ("Scale.Range:Maximum")) -> ()  [unwired: 2 in, 2 out]
            n95 = local write "Test Slider"(w159) -> ()
            n96 = property on="Motor" class="Clust (strict)"("Visible"=w158) -> ()  [unwired: 2 in, 2 out]
            n97 = property on="Rev/Fwd" class="Clust (strict)"("Visible"=w158) -> ()  [unwired: 2 in, 2 out]
            n98 = property on="On/Off" class="Bool (strict)"("Visible"=w158) -> ()  [unwired: 2 in, 2 out]
            n99 = property on="Test Ring" class="Ring (strict)"("Visible"=w158) -> ()  [unwired: 2 in, 2 out]
          }
          frame "Relay", "Solenoid" {
            w161 = FALSE ("Visible")
            n100 = property on="Motor" class="Clust (strict)"("Visible"=w161) -> ()  [unwired: 2 in, 2 out]
            n101 = property on="Test Slider" class="Slide (strict)"("Visible"=w161) -> ()  [unwired: 2 in, 2 out]
            n102 = Search and Replace String(input string=w162, search string="/Value  **", replace string="/Direction") -> (result string=w168:string)  [unwired: 5 in, 3 out]
            n103 = property on="Test Ring" class="Ring (strict)"("Visible"=w161) -> ()  [unwired: 2 in, 2 out]
            n104 = call <vilib>:"NT Read String.vi"("name"=w168) -> ("value"=w166:string)  [unwired: 8 in, 2 out]
            n105 = Equal?(x="Both directions", y=w166) -> (x = y?=w164:bool)
            n106 = Not(x=w164) -> (.not. x?=w165:bool)
            n107 = property on="Rev/Fwd" class="Clust (strict)"("Visible"=w164) -> ()  [unwired: 2 in, 2 out]
            n108 = property on="On/Off" class="Bool (strict)"("Visible"=w165, "Caption.Text"=w163) -> ()  [unwired: 2 in, 2 out]
          }
          frame "Compressor", "Digital Out" {
            w171 = FALSE ("Visible")
            # "Get direction and finish"
            n109 = property on="Motor" class="Clust (strict)"("Visible"=w171) -> ()  [unwired: 2 in, 2 out]
            n110 = property on="Test Slider" class="Slide (strict)"("Visible"=w171) -> ()  [unwired: 2 in, 2 out]
            n111 = property on="Test Ring" class="Ring (strict)"("Visible"=w171) -> ()  [unwired: 2 in, 2 out]
            n112 = property on="On/Off" class="Bool (strict)"("Visible"=TRUE, "Caption.Text"=w172) -> ()  [unwired: 2 in, 2 out]
            n113 = property on="Rev/Fwd" class="Clust (strict)"("Visible"=FALSE) -> ()  [unwired: 2 in, 2 out]
          }
          frame "Camera" {
            n114 = call <vilib>:"NT_Get Last Path Segment.vi"("String in"=w179) -> ("String out"=w180:string)  [unwired: 10 in]
            n115 = property on="On/Off" class="Bool (strict)"("Visible"=FALSE) -> ()  [unwired: 2 in, 2 out]
            n116 = property on="Motor" class="Clust (strict)"("Visible"=FALSE) -> ()  [unwired: 2 in, 2 out]
            n117 = property on="Rev/Fwd" class="Clust (strict)"("Visible"=FALSE) -> ()  [unwired: 2 in, 2 out]
            n118 = case shown="\"White Balance  **\"" w180 {
              tunnel: w179 -> [w186 w195 w204 w213 w222 _ w228]
              tunnel: w178 -> [w184 w192 w201 w210 w219 _ _]
              frame "Size  **" {
                n119 = Index Array(array=w184) -> (element=w183:cluster{string[]})  [unwired: 1 in]
                n120 = call <vilib>:"NT Read String.vi"("name"=w186) -> ("value"=w185:string)  [unwired: 8 in, 2 out]
                n121 = Unbundle(w183) -> (w181:string[])
                n122 = Match First String(2:w181, 3:w185) -> (0:w182:i32)  [unwired: 1 out]
                n123 = property on="Test Ring" class="Ring (strict)"("Value"=w182, "Strings []"=w181) -> ()  [unwired: 2 in, 2 out]
                n124 = property on="Test Ring" class="Ring (strict)"("Visible"=TRUE) -> ()  [unwired: 2 in, 2 out]
                n125 = property on="Test Slider" class="Slide (strict)"("Visible"=FALSE) -> ()  [unwired: 2 in, 2 out]
              }
              frame "White Balance  **" {
                n126 = Index Array(array=w192, index=1) -> (element=w193:cluster{string[]})
                n127 = call <vilib>:"NT Read String.vi"("name"=w195) -> ("value"=w194:string)  [unwired: 8 in, 2 out]
                n128 = Unbundle(w193) -> (w190:string[])
                n129 = Match First String(2:w190, 3:w194) -> (0:w189:i32)  [unwired: 1 out]
                n130 = property on="Test Ring" class="Ring (strict)"("Value"=w189, "Strings []"=w190) -> ()  [unwired: 2 in, 2 out]
                n131 = property on="Test Ring" class="Ring (strict)"("Visible"=TRUE) -> ()  [unwired: 2 in, 2 out]
                n132 = property on="Test Slider" class="Slide (strict)"("Visible"=FALSE) -> ()  [unwired: 2 in, 2 out]
              }
              frame "Exposure  **" {
                n133 = Index Array(array=w201, index=2) -> (element=w202:cluster{string[]})
                n134 = call <vilib>:"NT Read String.vi"("name"=w204) -> ("value"=w203:string)  [unwired: 8 in, 2 out]
                n135 = Unbundle(w202) -> (w198:string[])
                n136 = Match First String(2:w198, 3:w203) -> (0:w199:i32)  [unwired: 1 out]
                n137 = property on="Test Ring" class="Ring (strict)"("Value"=w199, "Strings []"=w198) -> ()  [unwired: 2 in, 2 out]
                n138 = property on="Test Ring" class="Ring (strict)"("Visible"=TRUE) -> ()  [unwired: 2 in, 2 out]
                n139 = property on="Test Slider" class="Slide (strict)"("Visible"=FALSE) -> ()  [unwired: 2 in, 2 out]
              }
              frame "Exposure Priority  **" {
                n140 = Index Array(array=w210, index=3) -> (element=w211:cluster{string[]})
                n141 = call <vilib>:"NT Read String.vi"("name"=w213) -> ("value"=w212:string)  [unwired: 8 in, 2 out]
                n142 = Unbundle(w211) -> (w207:string[])
                n143 = Match First String(2:w207, 3:w212) -> (0:w208:i32)  [unwired: 1 out]
                n144 = property on="Test Ring" class="Ring (strict)"("Value"=w208, "Strings []"=w207) -> ()  [unwired: 2 in, 2 out]
                n145 = property on="Test Ring" class="Ring (strict)"("Visible"=TRUE) -> ()  [unwired: 2 in, 2 out]
                n146 = property on="Test Slider" class="Slide (strict)"("Visible"=FALSE) -> ()  [unwired: 2 in, 2 out]
              }
              frame "Color Enable  **" {
                n147 = Index Array(array=w219, index=4) -> (element=w220:cluster{string[]})
                n148 = call <vilib>:"NT Read String.vi"("name"=w222) -> ("value"=w221:string)  [unwired: 8 in, 2 out]
                n149 = Unbundle(w220) -> (w216:string[])
                n150 = Match First String(2:w216, 3:w221) -> (0:w217:i32)  [unwired: 1 out]
                n151 = property on="Test Ring" class="Ring (strict)"("Value"=w217, "Strings []"=w216) -> ()  [unwired: 2 in, 2 out]
                n152 = property on="Test Ring" class="Ring (strict)"("Visible"=TRUE) -> ()  [unwired: 2 in, 2 out]
                n153 = property on="Test Slider" class="Slide (strict)"("Visible"=FALSE) -> ()  [unwired: 2 in, 2 out]
              }
              frame Default {
                n154 = property on="Test Ring" class="Ring (strict)"("Visible"=FALSE) -> ()  [unwired: 2 in, 2 out]
                n155 = property on="Test Slider" class="Slide (strict)"("Visible"=FALSE) -> ()  [unwired: 2 in, 2 out]
              }
              frame "Brightness  **", "Color Level  **", "Compression  **", "FPS  **", "Sharpness  **" {
                n156 = call <vilib>:"NT Read Number.vi"("name"=w228) -> ("value"=w227:dbl)  [unwired: 8 in, 2 out]
                n157 = local write "Test Slider"(w227) -> ()
                n158 = property on="Test Slider" class="Slide (strict)"("Visible"=TRUE, "Scale.Maximum"=100.0 ("Scale.Range:Maximum")) -> ()  [unwired: 2 in, 2 out]
                n159 = property on="Test Ring" class="Ring (strict)"("Visible"=FALSE) -> ()  [unwired: 2 in, 2 out]
              }
            }
          }
        }
        n160 = property on="Progress" class="Clust (strict)"("Visible"=FALSE) -> ()  [unwired: 2 in, 2 out]
      }
      event "Test Name": Mouse Enter {
        # "Populate the ring with the list of tests"
        n161 = event-data() -> ()  [unwired: 1 in, 1 out]
        n162 = call <vilib>:"NT Read String Array.vi"("name"="TestMode/TestList" ("Name")) -> ("value"=w235:string[])  [unwired: 8 in, 2 out]
        n163 = Build Array (concatenate)("Select the test to run...", w235) -> (w234:string[])
        n164 = property on="Test Name" class="Ring (strict)"("Strings []"=w234) -> ()  [unwired: 2 in, 2 out]
      }
      event "Test Name": Value Change {
        w236 = FALSE ("Visible")
        # "Tell the robot the test name to run"
        n165 = event-data() -> ("NewVal"=w240:u16)  [unwired: 1 in]
        n166 = property on="Test Name" class="Ring (strict)"() -> ("Strings []"=w241:string[])  [unwired: 2 in, 2 out]
        n167 = local write "Progress"(T8 {"Test Progress"=0, "Test Progress Text"=""} ("Progress")) -> ()
        n168 = Index Array(array=w241, index=w240) -> (element=w239:string)
        n169 = call <vilib>:"NT Write String.vi"("value"=w239, "name"="TestMode/TestName" ("Name")) -> ()  [unwired: 9 in, 1 out]
        n170 = property on="Progress" class="Clust (strict)"("Visible"=TRUE) -> ()  [unwired: 2 in, 2 out]
        n171 = property on="Motor" class="Clust (strict)"("Visible"=w236) -> ()  [unwired: 2 in, 2 out]
        n172 = property on="Test Slider" class="Slide (strict)"("Visible"=w236) -> ()  [unwired: 2 in, 2 out]
        n173 = property on="On/Off" class="Bool (strict)"("Visible"=w236) -> ()  [unwired: 2 in, 2 out]
        n174 = property on="Rev/Fwd" class="Clust (strict)"("Visible"=w236) -> ()  [unwired: 2 in, 2 out]
        n175 = property on="Test Ring" class="Ring (strict)"("Visible"=w236) -> ()  [unwired: 2 in, 2 out]
      }
      event "CheckList": Double Click {
        # "Shift clears all"
        # "Update symbols on the listbox"
        n176 = event-data() -> ("PlatMods.Shift"=w243:bool, "Row"=w245:i32)  [unwired: 1 in]
        n177 = case shown="True" w243 {
          tunnel: w245 -> [w249 _]
          tunnel: 1 -> [w248 _]
          frame False {
            n178 = property on="CheckList" class="LstBox (strict)"() -> ("Item Symbols"=w247:i32[])  [unwired: 2 in, 2 out]
            n179 = Replace Array Subset(array=w247, new element=w248, index=w249) -> (w246:i32[])
            n180 = property on="CheckList" class="LstBox (strict)"("Item Symbols"=w246) -> ()  [unwired: 2 in, 2 out]
          }
          frame True {
            w250 = 0 ("Top Row")
            n181 = property on="CheckList" class="LstBox (strict)"() -> ("Number of Rows"=w252:u32)  [unwired: 2 in, 2 out]
            n182 = Initialize Array(0, w252) -> (w251:i32[])
            n183 = property on="CheckList" class="LstBox (strict)"("Top Row"=w250, "Value"=w250, "Item Symbols"=w251) -> ()  [unwired: 2 in, 2 out]
          }
        }
      }
      event "CheckList": Key Down {
        # "Update symbols on the listbox\nLeft and right keys check and uncheck"
        n184 = event-data() -> ("VKey"=w255:T17)  [unwired: 1 in]
        n185 = case shown="\"Left\", \"Right\"" w255 {
          selector: w255 -> [w260 _]
          tunnel: eventvkey."Left" ("VKey") -> [w258 _]
          frame "Left", "Right" {
            n186 = Equal?(x=w258, y=w260) -> (x = y?=w259:bool)
            n187 = Select(t=0, s=w259, f=1) -> (s? t:f=w261:i32)
            n188 = property on="CheckList" class="LstBox (strict)"() -> ("Item Symbols"=w264:i32[])  [unwired: 2 in, 2 out]
            n189 = Replace Array Subset(array=w264, new element=w261, index="CheckList") -> (w263:i32[])
            n190 = property on="CheckList" class="LstBox (strict)"("Item Symbols"=w263) -> ()  [unwired: 2 in, 2 out]
          }
          frame Default {
          }
        }
      }
      event "Motor.Enable": Value Change {
        # "When the test mode otor enable helper is set, update that\ntree row item's value"
        n191 = event-data() -> ("NewVal"=w269:bool)  [unwired: 1 in]
        n192 = Unbundle("Motor") -> ("Value"=w268:dbl)  [unwired: 1 out]
        n193 = Select(t=w268, s=w269, f=0.0) -> (s? t:f=w266:dbl)
        n194 = call <vilib>:"NT Write Number.vi"("value"=w266, "name"=w265) -> ()  [unwired: 9 in, 1 out]
      }
      event "Test Slider": Value Change {
        # "When the test mode slider helper is set, update that\ntree row item's value"
        n195 = event-data() -> ("NewVal"=w271:dbl)  [unwired: 1 in]
        n196 = call <vilib>:"NT Write Number.vi"("value"=w271, "name"=w272) -> ()  [unwired: 9 in, 1 out]
      }
      event "On/Off": Value Change {
        # "When the test mode on/off helper value is set, update that\ntree row item's value"
        n197 = event-data() -> ("NewVal"=w275:bool)  [unwired: 1 in]
        n198 = Boolean To (0,1)(Boolean=w275) -> (0, 1=w274:i16)
        n199 = call <vilib>:"NT Write Number.vi"("value"=w274, "name"=w273) -> ()  [unwired: 9 in, 1 out]
      }
      event "Rev/Fwd": Value Change {
        # "When the test mode helper value for relays is set, update that\ntree row item's value"
        n200 = event-data() -> ("NewVal.Forward"=w282:bool, "NewVal.Reverse"=w281:bool)  [unwired: 1 in]
        n201 = Boolean To (0,1)(Boolean=w282) -> (0, 1=w278:i16)
        n202 = Boolean To (0,1)(Boolean=w281) -> (0, 1=w280:i16)
        n203 = Negate(x=w280) -> (-x=w279:i16)
        n204 = Add(x=w278, y=w279) -> (x+y=w277:i16)
        n205 = call <vilib>:"NT Write Number.vi"("value"=w277, "name"=w276) -> ()  [unwired: 9 in, 1 out]
      }
      event "Test Ring": Value Change {
        # "When a test mode helper value is selected from the ring,\nset the tree item's variable to the string value"
        n206 = event-data() -> ("NewVal"=w285:u16)  [unwired: 1 in]
        n207 = property on="Test Ring" class="Ring (strict)"() -> ("Strings []"=w286:string[])  [unwired: 2 in, 2 out]
        n208 = Index Array(array=w286, index=w285) -> (element=w284:string)
        n209 = call <vilib>:"NT Write String.vi"("value"=w284, "name"=w283) -> ()  [unwired: 9 in, 1 out]
      }
      event "Rec Mode": Value Change {
        # "Update globals for recording mode and path to read log from.\nClear when logging and let NetworkTables set path for vision to\nuse."
        n210 = event-data() -> ("NewVal"=w295:enum32{"Stop", "Record", "Playback"})  [unwired: 1 in]
        n211 = global write "WPI_DashboardLogging Global.vi" "Logging Filename"(path "") -> ()
        n212 = global write "WPI_DashboardLogging Global.vi" "Recording"(w295) -> ()
        n213 = case shown="\"Playback\"" w295 {
          tunnel: w294 -> [_ w297 w305]
          tunnel: [_ _ w304] -> w292
          tunnel: [_ _ w303] -> _
          tunnel: w290 -> [_ _ w301]
          tunnel: cluster{i32, i32} {-250, 170} -> [_ _ w300]
          tunnel: [_ _ T18 {"Image Size"=TRUE, "Image Type"=TRUE, "Pixel Value"=TRUE, "ROI Information"=TRUE, "Zoom Factor"=FALSE} ("Image Information Shown:All Elements")] -> w287
          tunnel: [_ _ TRUE ("Zoom Factor")] -> w288
          frame Default {
          }
          frame "Stop", "Record" {
            # "Place Window too"
            n214 = invoke class="VI" method="FP.Close"(reference=w297) -> (reference out=w296:refnum<vi>)  [unwired: 2 in, 2 out]
            n215 = invoke class="VI" method="Abort VI"(reference=w296) -> ()  [unwired: 2 in, 3 out]
          }
          frame "Playback" {
            n216 = call "Open Playback Panel.vi"("Offset"=w300, "DB VI Ref"=w301, "Playback in"=w305) -> ("Playback out"=w302:refnum<vi>)  [unwired: 8 in]
            n217 = register-events(w302) -> (reference out=w304:refnum<event-registration>, error out=w303:errorcluster)  [unwired: 2 in]
          }
        }
        n218 = property on="Camera Image" class="ImageControl"("Image Information Shown"=w287, "Image Information Visible"=w288) -> ()  [unwired: 2 in, 2 out]
        n219 = call <vilib>:"WPI_DashboardNT Log FieldName Cache.vi"("Operation"=enum16{"Lookup/Add", "Index", "Clear"}."Clear") -> ()  [unwired: 8 in, 3 out]
      }
      event Panel Close {
        w306 = enum32{"Stop", "Record", "Playback"}."Stop" ("Rec Mode")
        # "Playback window has been closed, abort"
        n220 = event-data() -> ()  [unwired: 1 in, 4 out]
        n221 = local write "Rec Mode"(w306) -> ()
        n222 = global write "WPI_DashboardLogging Global.vi" "Recording"(w306) -> ()
      }
      event Panel Close {
        # "Abort playback window and ourself"
        n223 = event-data() -> ()  [unwired: 1 in, 4 out]
        n224 = invoke class="VI" method="FP.Close"(reference=w309) -> (reference out=w308:refnum<vi>)  [unwired: 2 in, 2 out]
        n225 = invoke class="VI" method="Abort VI"(reference=w308) -> (error out=w307:errorcluster)  [unwired: 2 in, 2 out]
        n226 = invoke class="VI" method="Abort VI"(error in=w307) -> ()  [unwired: 2 in, 3 out]
      }
      event "Tree": Double Click {
        n227 = event-data() -> ("PlatMods"=w315:T20, "Tag"=w312:string)  [unwired: 1 in]
        n228 = Unbundle(w315) -> ("Shift"=w314:bool)  [unwired: 4 out]
        n229 = String Subset(string=w312, length (rest)=1 ("length (rest)")) -> (substring=w311:string)  [unwired: 1 in]
        n230 = Not(x=w314) -> (.not. x?=w313:bool)
        n231 = case shown="\"/\"" w311 {
          tunnel: w312 -> [_ w317]
          tunnel: w313 -> [_ w316]
          frame Default {
          }
          frame "/" {
            n232 = call <vilib>:"NT Update Persistence.vi"("Persistence"=w316, "Name"=w317) -> ()  [unwired: 9 in, 1 out]
          }
        }
      }
    }
  }
  n233 = while {
    tunnel: w50 -> [w319]
    i -> [w322]
    stop <- FALSE stop-if-true
    n234 = Wait (ms)(milliseconds to wait=u32 100) -> ()  [unwired: 1 out]
    n235 = case shown="\"Playback\"" "Rec Mode" {
      tunnel: w322 -> [_ _ w337]
      tunnel: [u32 2829099 ("Base Color") u32 11141120 ("Target Color") w326] -> w318
      frame "Stop", Default {
        # "Reset the color, extra updates don't cost much"
      }
      frame "Record" {
      }
      frame "Playback" {
        # "Playback"
        n236 = Quotient & Remainder(x=w337, y=u32 50 ("milliseconds to wait")) -> (x-y*floor(x/y)=w333:u32)  [unwired: 1 out]
        n237 = Divide(x=w333, y=u32 50 ("milliseconds to wait")) -> (x/y=w330:dbl)
        n238 = Multiply(x=6.283185307179586, y=w330) -> (x*y=w335:dbl)
        n239 = Sine(x=w335) -> (sin(x)=w334:dbl)
        n240 = Absolute Value(x=w334) -> (abs(x)=w327:dbl)
        n241 = call "Interpolate RGB Color.vi"("Proportion"=w327, "Target Color"=u32 30976, "Base Color"=u32 2829099) -> ("Result Color"=w326:u32)  [unwired: 8 in]
      }
    }
    n242 = property class="Pane"(reference=w319, "PaneColor"=w318) -> ()  [unwired: 1 in, 2 out]
  }
  n243 = local write "Dashboard Tab"(T3."Drive" ("Dashboard Tab")) -> ()
  n244 = property on="On/Off" class="Bool (strict)"("Visible"=w25) -> ()  [unwired: 2 in, 2 out]
  n245 = property on="Motor" class="Clust (strict)"("Visible"=w25) -> ()  [unwired: 2 in, 2 out]
  n246 = property on="Progress" class="Clust (strict)"("Visible"=w25) -> ()  [unwired: 2 in, 2 out]
  n247 = property on="Test Ring" class="Ring (strict)"("Visible"=w25) -> ()  [unwired: 2 in, 2 out]
  n248 = property on="Rev/Fwd" class="Clust (strict)"("Visible"=w25) -> ()  [unwired: 2 in, 2 out]
  n249 = while {
    tunnel: u16 1741 ("timeout ms (25000)") -> [w339]
    stop <- FALSE stop-if-true
    n250 = TCP Create Listener(10:w339) -> (0:w338:errorcluster, 3:w340:refnum<k5>)  [unwired: 4 in, 1 out]
    n251 = case shown="No Error" w338 {
      selector: w338 -> [w342 _]
      tunnel: w340 -> [w343 _]
      frame No Error {
        n252 = while {
          tunnel: w343 -> [w346]
          tunnel: w342 -> [w345]
          stop <- FALSE stop-if-true
          n253 = TCP Wait On Listener(8:w345, 11:w346) -> (0:w347:errorcluster, 4:w348:refnum<k5>)  [unwired: 2 in, 3 out]
          n254 = local write "TCP"(w348) -> ()
          n255 = case shown="Error" w347 {
            frame No Error {
            }
            frame Error {
              n256 = Wait (ms)(milliseconds to wait=u32 1000) -> ()  [unwired: 1 out]
            }
          }
        }
      }
      frame Error {
        n257 = Wait (ms)(milliseconds to wait=u32 1000) -> ()  [unwired: 1 out]
      }
    }
  }
  n258 = global write "WPI_DashboardLogging Global.vi" "Recording"(w45) -> ()
  n259 = local write "Rec Mode"(w45) -> ()
  n260 = property on="Current" class="DigNum (strict)"("NumText.BG Color"=w2, "NumText.BGColor"=w2) -> ()  [unwired: 2 in, 2 out]
  n261 = control-ref of="Field Picture"() -> (w10:refnum<vi>)
  n262 = control-ref of="ROBOT"() -> (w12:refnum<vi>)
  n263 = control-ref of="Field Picture"() -> (w13:refnum<vi>)
  n264 = call <vilib>:"FieldDisp_Element_Prepare.vi"("Element File Name"="Robot_kitbot_5.png" ("Picture FIle Name"), "Element Picture Ref"=w12, "Field Picture Ref"=w13) -> ("Field Element Info"=w5:T21)  [unwired: 7 in, 1 out]
  n265 = call <vilib>:"FieldDisp_Field_Disp.vi"("Field Selector"="2023 Charged Up", "Picture in"=w10) -> ("error out"=w8:errorcluster)  [unwired: 9 in]
  n266 = while {
    tunnel: [w360] -> _
    tunnel: w24 -> [w352]
    tunnel: w8 -> [_]
    tunnel: w5 -> [w351]
    i -> [w360]
    stop <- FALSE stop-if-true
    n267 = call <vilib>:"WPI_DashboardRetrieveStatusInfo.vi"("Window Mode Notifier"=w352, "TCP Cnx"="TCP") -> ("Power and Errors"=w355:T22, "Robot Metrics"=w358:T23, "Status Info"=w359:T24, "Control Info"=w356:T25, "Robot Mode"=w354:T5, "Process?"=w357:bool)  [unwired: 4 in]
    "Mode" <- w354
    n268 = case shown="True" w357 {
      tunnel: w359 -> [_ w444]
      tunnel: w358 -> [_ w443]
      tunnel: w356 -> [_ _]
      tunnel: w355 -> [_ w442]
      tunnel: w354 -> [_ _]
      tunnel: w351 -> [_ w404]
      frame False {
        n269 = Wait (ms)(milliseconds to wait=u32 20) -> ()  [unwired: 1 out]
      }
      frame True {
        w366 = WPI_SolenoidValue."Off" ("Value")
        w373 = WPI_SolenoidValue."Off" ("Value")
        # "Double Solenoid"
        # "Single Solenoid"
        # "Compressor"
        # "tab changed."
        # "y"
        # "x"
        n270 = Unbundle By Name(w443) -> ()  [unwired: 1 out]
        n271 = Unbundle By Name(w442) -> ("Robot IP"=→"Robot IP":string)
        n272 = Unbundle By Name(w444) -> ()  [unwired: 2 out]
        n273 = call-poly <vilib>:"NT Write Value.vi"("value"="Distance", "name"="Auto/QuickDistance") -> ()  [unwired: 9 in, 1 out]
        n274 = call-poly <vilib>:"NT Write Value.vi"("value"="Position", "name"="Auto/QuickPosition") -> ()  [unwired: 9 in, 1 out]
        n275 = call-poly <vilib>:"NT Write Value.vi"("value"="Game Piece", "name"="Auto/QuickGamePiece") -> ()  [unwired: 9 in, 1 out]
        n276 = call-poly <vilib>:"NT Read Value.vi"("name"="Sol-2-output") -> ("value"=w365:i64)  [unwired: 8 in, 2 out]
        n277 = call-poly <vilib>:"NT Read Value.vi"("name"="Sol-1-output") -> ("value"=w372:i64)  [unwired: 8 in, 2 out]
        n278 = Coerce To Type(0:w365, 1:w366) -> (2:→"Double Cmd1":T4)
        n279 = Type Cast(type=w366, x=w365) -> (*(type *) &x=→"Double Cmd2":T4)
        n280 = Coerce To Type(0:w372, 1:w373) -> (2:→"Single Cmd1":T4)
        n281 = Type Cast(type=w373, x=w372) -> (*(type *) &x=→"Single Cmd2":T4)
        n282 = call-poly <vilib>:"NT Read Value.vi"("name"="LS2") -> ("value"=→"Request":bool)  [unwired: 8 in, 2 out]
        n283 = call-poly <vilib>:"NT Read Value.vi"("name"="LS1") -> ("value"=→"Request":bool)  [unwired: 8 in, 2 out]
        n284 = call-poly <vilib>:"NT Read Value.vi"("name"="Vision/Left vision found count") -> ("value"=w394:dbl)  [unwired: 8 in, 2 out]
        n285 = call-poly <vilib>:"NT Read Value.vi"("name"="Vision/Right vision found count") -> ("value"=w390:dbl)  [unwired: 8 in, 2 out]
        n286 = feedback-in #1(w394) -> ()
        n287 = feedback #1() -> (w393:dbl)  [unwired: 1 in]
        n288 = feedback #2() -> (w389:dbl)  [unwired: 1 in]
        n289 = feedback-in #2(w390) -> ()
        n290 = call-poly <vilib>:"NT Read Value.vi"("name"="Vision/Left vision connect") -> ("value"=→"Left Cam Connected":bool)  [unwired: 8 in, 2 out]
        n291 = call-poly <vilib>:"NT Read Value.vi"("name"="Vision/Right vision connect") -> ("value"=→"Right Cam Connected":bool)  [unwired: 8 in, 2 out]
        n292 = Not Equal?(x=w394, y=w393) -> (x != y?=→"Left April Tag Updated":bool)
        n293 = Not Equal?(x=w390, y=w389) -> (x != y?=→"Right April Tag Updated":bool)
        n294 = call-poly <vilib>:"NT Read Value.vi"("name"="Compressor/Enabled") -> ("value"=→"Enabled":bool)  [unwired: 8 in, 2 out]
        n295 = call-poly <vilib>:"NT Read Value.vi"("name"="Compressor/Current") -> ("value"=→"Current":dbl)  [unwired: 8 in, 2 out]
        n296 = call-poly <vilib>:"NT Read Value.vi"("name"="Compressor/Running") -> ("value"=→"Running":bool)  [unwired: 8 in, 2 out]
        n297 = case shown="True" "Update" {
          tunnel: "Starting X Ft" -> [_ w461]
          tunnel: "Starting Y Ft" -> [_ w460]
          tunnel: "Starting Heading Deg" -> [_ w459]
          frame False {
          }
          frame True {
            n298 = call-poly <vilib>:"NT Write Value.vi"("value"=w461, "name"="Vision/X initial in feet DASH") -> ()  [unwired: 9 in, 1 out]
            n299 = call-poly <vilib>:"NT Write Value.vi"("value"=w459, "name"="Vision/angle initial DASH") -> ()  [unwired: 9 in, 1 out]
            n300 = call-poly <vilib>:"NT Write Value.vi"("value"=w460, "name"="Vision/Y initial in feet DASH") -> ()  [unwired: 9 in, 1 out]
          }
        }
        n301 = call-poly <vilib>:"NT Read Value.vi"("name"="Vision/Xcurrent in feet") -> ("value"=w402:dbl)  [unwired: 8 in, 2 out]
        "Odom X Pos Ft" <- w402
        n302 = call-poly <vilib>:"NT Read Value.vi"("name"="Vision/Y current in feet") -> ("value"=w386:dbl)  [unwired: 8 in, 2 out]
        "Odom Y Pos Ft" <- w386
        n303 = call-poly <vilib>:"NT Read Value.vi"("name"="Vision/angle current") -> ("value"=w387:dbl)  [unwired: 8 in, 2 out]
        "Odom Heading Deg" <- w387
        n304 = local read "Dashboard Tab"() -> (w383:T3)
        n305 = call <vilib>:"Conv_Feet_Meters.vi"("Feet"=w402) -> ("Meters"=w401:dbl)  [unwired: 10 in]
        n306 = call <vilib>:"Conv_Feet_Meters.vi"("Feet"=w386) -> ("Meters"=w400:dbl)  [unwired: 10 in]
        n307 = call <vilib>:"Conv_Deg_Radians.vi"("Degress"=w387) -> ("Radians"=w403:dbl)  [unwired: 10 in]
        n308 = Equal?(x=T10."Field" ("Dashboard Tab"), y=w383) -> (x = y?=w385:bool)
        n309 = feedback-in #3(w383) -> ()
        n310 = feedback #3() -> (w382:T3)  [unwired: 1 in]
        n311 = Not Equal?(x=w383, y=w382) -> (x != y?=w381:bool)
        n312 = case shown="True" w385 {
          tunnel: w404 -> [w446 w451]
          tunnel: w403 -> [_ w454]
          tunnel: w401 -> [_ w453]
          tunnel: w400 -> [_ w452]
          tunnel: w381 -> [w445 w450]
          frame False {
            n313 = case shown="True" w445 {
              tunnel: w446 -> [_ w447]
              frame False {
              }
              frame True {
                n314 = Unbundle By Name(w447) -> ("Element Picture Ref"=w448:refnum<vi>)
                n315 = property class="Pict"(reference=w448, "Visible"=FALSE) -> ()  [unwired: 1 in, 2 out]
              }
            }
          }
          frame True {
            # "Update display\nof field element\n(robot)"
            n316 = call <vilib>:"Pose2d_New.vi"("Heading"=w454, "Y"=w452, "X"=w453) -> ("out POSe"=w455:T26)  [unwired: 8 in]
            n317 = call <vilib>:"FieldDisp_Element_Disp.vi"("Element Pose"=w455, "Element Info"=w451) -> ()  [unwired: 10 in]
            n318 = case shown="True" w450 {
              tunnel: w451 -> [_ w456]
              frame False {
              }
              frame True {
                n319 = Unbundle By Name(w456) -> ("Element Picture Ref"=w457:refnum<vi>)
                n320 = property class="Pict"(reference=w457, "Visible"=TRUE) -> ()  [unwired: 1 in, 2 out]
              }
            }
          }
        }
        n321 = call-poly <vilib>:"NT Read Value.vi"("name"="drive/LSpeedDem") -> ("value"=w431:dbl)  [unwired: 8 in, 2 out]
        n322 = call-poly <vilib>:"NT Read Value.vi"("name"="drive/LeftSpeed") -> ("value"=w430:dbl)  [unwired: 8 in, 2 out]
        n323 = call-poly <vilib>:"NT Read Value.vi"("name"="drive/LeftMotorOutput") -> ("value"=w429:dbl)  [unwired: 8 in, 2 out]
        n324 = call-poly <vilib>:"NT Read Value.vi"("name"="drive/RSpeedDem") -> ("value"=w425:dbl)  [unwired: 8 in, 2 out]
        n325 = call-poly <vilib>:"NT Read Value.vi"("name"="drive/RightSpeed") -> ("value"=w424:dbl)  [unwired: 8 in, 2 out]
        n326 = call-poly <vilib>:"NT Read Value.vi"("name"="drive/RightMotorOutput") -> ("value"=w423:dbl)  [unwired: 8 in, 2 out]
        n327 = call-poly <vilib>:"NT Read Value.vi"("name"="Arm/ExtendDmd") -> ("value"=w419:dbl)  [unwired: 8 in, 2 out]
        n328 = call-poly <vilib>:"NT Read Value.vi"("name"="Arm/ExtendPos") -> ("value"=w418:dbl)  [unwired: 8 in, 2 out]
        n329 = call-poly <vilib>:"NT Read Value.vi"("name"="Arm/ExtendMotOut") -> ("value"=w417:dbl)  [unwired: 8 in, 2 out]
        n330 = Bundle("value"=w431, "value"=w430, "value"=w429) -> (→"Compressor Chart":cluster{"value":dbl, "value":dbl, "value":dbl})  [unwired: 1 in]
        n331 = Bundle("value"=w425, "value"=w424, "value"=w423) -> (→"Single Solenoid Chart":cluster{"value":dbl, "value":dbl, "value":dbl})  [unwired: 1 in]
        n332 = Bundle("value"=w419, "value"=w418, "value"=w417) -> (→"Double Solenoid Chart":cluster{"value":dbl, "value":dbl, "value":dbl})  [unwired: 1 in]
      }
    }
  }
